vi "Error Logger.vi"(8 "error in":errorcluster, 9 "VI_name":string, 10 "Error":errorcluster, 11 "Case":string) -> (0 "error out":errorcluster)   [LabVIEW 2024]
uses:
  Launcher/Launcher_DTU.lvlib
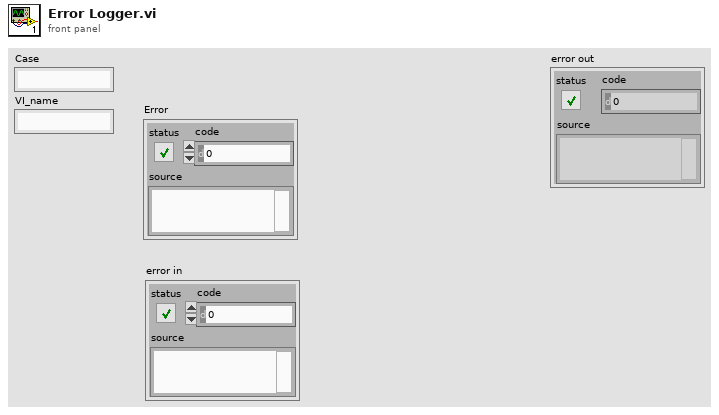
[diagram p1: front panel]
types:
  T1 = enum16{"open", "replace", "create", "open or create", "replace or create", "replace or create with confirmation"}
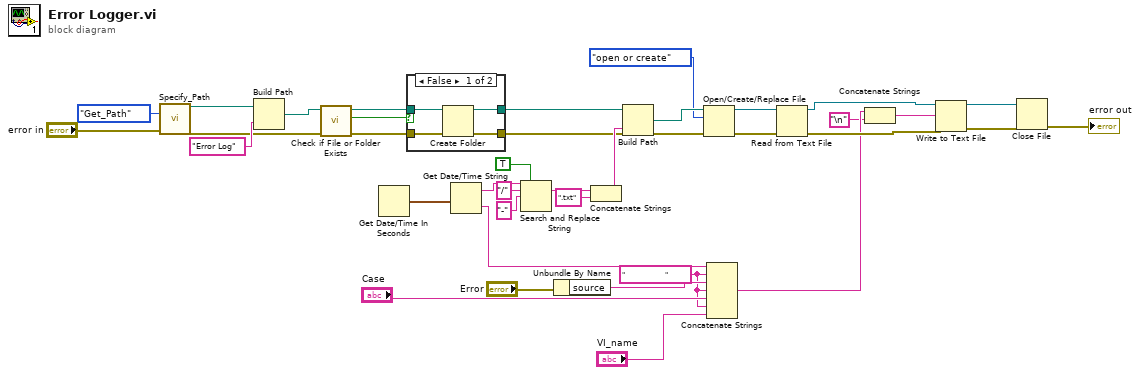
[diagram p0: block diagram]
diagram:
  w12 = "                    " ("string")
  n1 = call "Specify_Path.vi"("Path_Enum"=enum16{"Find_Path", "Get_Path"}."Get_Path", "error in (no error)"="error in") -> ("Configurations"=w30:path, "error out"=w26:errorcluster)  [unwired: 6 in, 6 out]
  n2 = Build Path(base path=w30, name or relative path="Error Log") -> (appended path=w28:path)
  n3 = call <vilib>:"Check if File or Folder Exists.vi"("error in (no error)"=w26, "path"=w28) -> ("error out"=w25:errorcluster, "file or folder exists?"=w27:bool, "dup path"=w24:path)  [unwired: 7 in]
  n4 = Get Date/Time In Seconds() -> (seconds since 1Jan1904=w37:timestamp)
  n5 = case shown="False" w27 {
    tunnel: w25 -> [w41 w42]
    tunnel: w24 -> [w40 w43]
    tunnel: [w39 w42] -> w21
    tunnel: [w38 w43] -> w23
    frame False {
      n6 = Create Folder(path (use dialog)=w40, error in=w41) -> (created path=w38:path, error out=w39:errorcluster)  [unwired: 1 in, 1 out]
    }
    frame True {
    }
  }
  n7 = Get Date/Time String(seconds (now)=w37) -> (date string=w34:string, time string=w15:string)  [unwired: 2 in]
  n8 = Search and Replace String(replace all?=TRUE ("replace all? (F)"), input string=w34, search string="/", replace string="-" ("replace string (\"\")")) -> (result string=w35:string)  [unwired: 4 in, 3 out]
  n9 = Unbundle By Name("Error") -> ("source"=w14:string)
  n10 = Concatenate Strings(w35, ".txt" ("string")) -> (w22:string)
  n11 = Build Path(base path=w23, name or relative path=w22) -> (appended path=w20:path)
  n12 = Open/Create/Replace File(file path (use dialog)=w20, error in=w21, operation (0:open)=T1."open or create") -> (refnum out=w4:refnum<file>, error out=w18:errorcluster)  [unwired: 3 in, 1 out]
  n13 = Concatenate Strings(w15, w12, w14, w12, "Case", w12, "VI_name") -> (w2:string)
  n14 = Read from Text File(file (use dialog)=w4, error in=w18) -> (refnum out=w3:refnum<file>, error out=w5:errorcluster)  [unwired: 2 in, 2 out]
  n15 = Concatenate Strings(w2, "\n") -> (w10:string)
  n16 = Write to Text File(file (use dialog)=w3, text=w10, error in=w5) -> (refnum out=w8:refnum<file>, error out=w9:errorcluster)  [unwired: 1 in, 1 out]
  n17 = Close File(refnum=w8, error in=w9) -> (error out=→"error out":errorcluster)  [unwired: 1 out]
